vi "Write Log Line.vi"(10 "Cluster":T1 {"Decoded Sensor Data"."Value" scale=0.0..10.0}, 11 "Byte Stream File in":refnum<file>) -> (3 "Byte Stream File out":refnum<file>)   [LabVIEW 2015]
uses:
  Telemetry Packet Type.ctl
  Thermocouple Data.ctl
  Sensors/Transducer Calibration Display.ctl
  Sensors/Sensor Enum.ctl
  Sequence Execution/Sequence Global Action.ctl
  Sequence Execution/Clock Control Enum.ctl
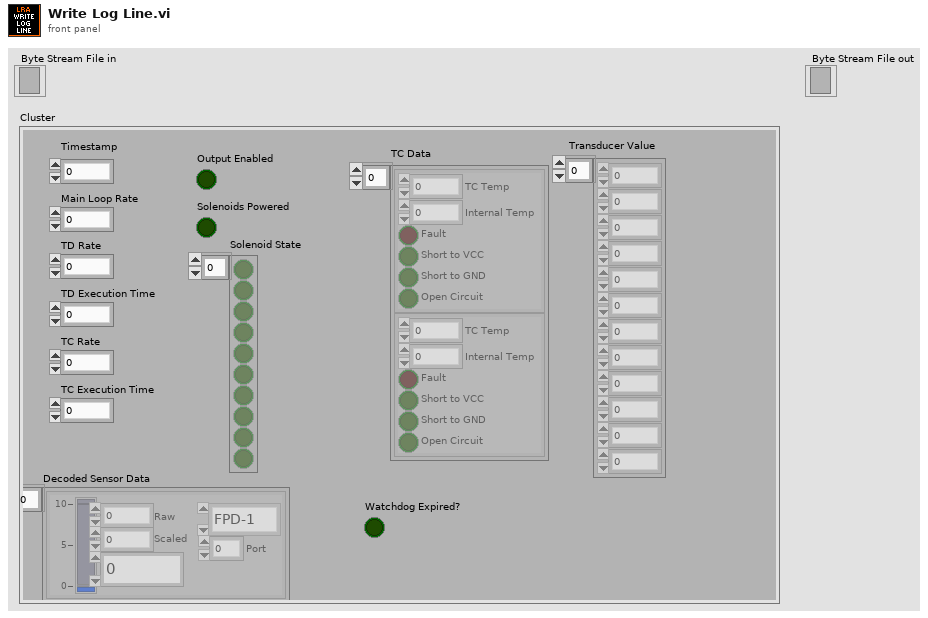
[diagram p1: front panel]
types:
  T1 = typedef "Telemetry Packet Type.ctl" = cluster{"Timestamp\n":u32, "Transducer Value":u16[], "Main Loop Rate":u32, "Solenoid State":bool[], "Output Enabled":bool, "Solenoids Powered":bool, "TC Data":T2[], "TD Rate":u32, "TD Execution Time":u32, "TC Rate":u32, "TC Execution Time":u32, "Decoded Sensor Data":T3[], "Watchdog Expired?":bool}
  T2 = typedef "Thermocouple Data.ctl" = cluster{"TC Temp":dbl, "Internal Temp":dbl, "Fault":bool, "Short to VCC":bool, "Short to GND":bool, "Open Circuit":bool}
  T3 = typedef "Transducer Calibration Display.ctl" = cluster{"Value":dbl, "Raw":dbl, "Scaled":dbl, "Sensor Name":T4, "Port":u32}
  T4 = typedef "Sensor Enum.ctl" = enum16{"FPD-1", "FPD-2", "FPD-3", "OPD-1", "OPD-2", "OPD-3", "AP-1", "PC-1", "PC-2", "VBAT", "VCOMP", "ICOMP", "TC-1", "TC-COMP"}
  T5 = typedef "Clock Control Enum.ctl" = enum16{"Set", "Get", "Start", "Stop", "Sequence Init"}
  T6 = typedef "Sequence Global Action.ctl" = enum16{"Get", "Set List", "Set Current"}
  T7 = typedef "Single Test Sequence.ctl" = cluster{"Actions":T8[], "Triggers":T11[], "Name":string}
  T8 = typedef "Test Sequence Action.ctl" = cluster{"Time":i32, "Action":T9, "Valve":T10}
  T9 = typedef "Valve Action Enum.ctl" = enum16{"Open", "Close"}
  T10 = typedef "Valve Name Enum.ctl" = enum16{"FV-2", "FV-3", "FV-4", "OV-2", "OV-3", "OV-4", "NV-2", "COMP"}
  T11 = typedef "Test Sequence Trigger.ctl" = cluster{"Sensor":T4, "Begin Time (ms)":u32, "End Time(ms)":u32, "Min Value":dbl, "Max Value":dbl, "Exceed Action":string}
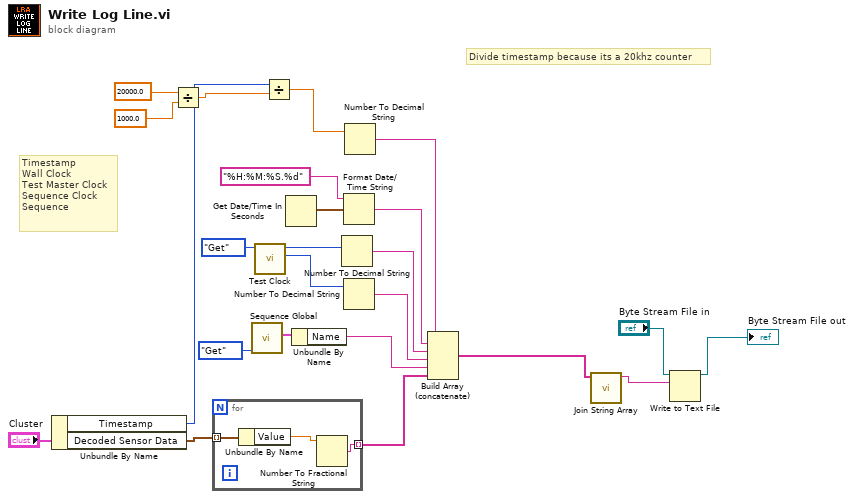
[diagram p0: block diagram]
diagram:
  # "Divide timestamp because its a 20khz counter"
  # "Timestamp\nWall Clock\nTest Master Clock\nSequence Clock\nSequence"
  n1 = Unbundle By Name("Cluster") -> ("Timestamp"=w5:u32, "Decoded Sensor Data"=w21:T3[])
  n2 = Divide(x=20000.0 ("y"), y=1000.0) -> (x/y=w1:dbl)
  n3 = for {
    tunnel: w21 -> [w27] mode=indexing
    tunnel: [w25] -> w9 mode=indexing
    n4 = Unbundle By Name(w27) -> ("Value"=w26:dbl)
    n5 = Number To Fractional String(number=w26) -> (F-format string=w25:string)  [unwired: 3 in]
  }
  n6 = call "Sequence Global.vi"("Action"=Sequence_Global_Action."Get") -> ("Current Sequence"=w14:T7)  [unwired: 8 in, 2 out]
  n7 = call "Test Clock.vi"("Command"=Clock_Control_Enum."Get") -> ("Time in Sequence"=w16:i32, "Master Time"=w17:i32)  [unwired: 8 in, 1 out]
  n8 = Divide(x=w5, y=w1) -> (x/y=w4:dbl)
  n9 = Get Date/Time In Seconds() -> (seconds since 1Jan1904=w19:timestamp)
  n10 = Unbundle By Name(w14) -> ("Name"=w10:string)
  n11 = Number To Decimal String(number=w17) -> (decimal integer string=w12:string)  [unwired: 1 in]
  n12 = Format Date/Time String(time format string (%c)="%H:%M:%S.%d", seconds (now)=w19) -> (date/time string=w13:string)  [unwired: 1 in]
  n13 = Number To Decimal String(number=w16) -> (decimal integer string=w11:string)  [unwired: 1 in]
  n14 = Number To Decimal String(number=w4) -> (decimal integer string=w6:string)  [unwired: 1 in]
  n15 = Build Array (concatenate)(w6, w13, w12, w11, w10, w9) -> (w8:string[])
  n16 = call "Join String Array.vi"("Array"=w8) -> ("String"=w22:string)  [unwired: 10 in]
  n17 = Write to Text File(file (use dialog)="Byte Stream File in", text=w22) -> (refnum out=→"Byte Stream File out":refnum<file>)  [unwired: 2 in, 2 out]
